vi "数据库加密匹配 (子VI).vi"(11 "输入参数":string) -> (3 "Encoded String":string)   [LabVIEW 2016, in "数据传输系统-04.lvlib"]
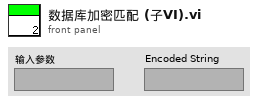
[diagram p1: front panel]
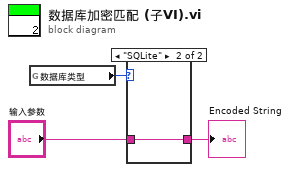
[diagram p0: block diagram]
diagram:
  n1 = global read "断电保存全局.vi" "数据库类型"() -> (w1:enum16{"Access", "SQLite"})
  n2 = case shown="\"SQLite\"" w1 {
    tunnel: "输入参数" -> [w4 w5]
    tunnel: [w4 w5] -> w3
    frame "Access", Default {
    }
    frame "SQLite" {
    }
  }
  "Encoded String" <- w3
